vi "GblVariableForLogging.vi"() -> ()   [LabVIEW 2019]
panel:
  in  "DataForLogging":dbl[](array[numeric])
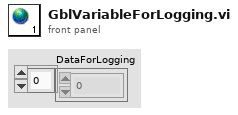
[diagram p1: front panel]
diagram:
